vi "Loop.vi"(9 "Error Queue":refnum<queue>, 10 "Helper Loop Queue":refnum<queue>, 11 "Dev Actor Panel":refnum<class "Dev Panel.lvclass">) -> ()   [LabVIEW 2021, in "Dev Panel.lvclass"]
uses:
  Dev Panel.lvclass
  C:/git/jettl/src/Event Actor/Event Actor.lvclass
  Event Actor/Event Actor.lvclass
  Dev Panel.lvclass/Dev Panel.ctl
  Actor/Msgs/Teardown/Teardown Msg/Teardown Msg.lvclass
  C:/git/jettl/src/Actor/Msg/Msg.lvclass
  Msgs/Pop Up/Pop Up Msg/Pop Up Msg.lvclass
  Actor/Msgs/Merge Error/Merge Error Msg/Merge Error Msg.lvclass
panel:
  in  "Button":bool
  out "String Indicator":string
  in  "Pop Up":bool
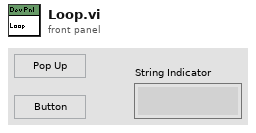
[diagram p1: front panel]
types:
  T1 = cluster{"Teardown":refnum<user-event>, "Pop Up":refnum<user-event>, "String Indicator":refnum<user-event>, "Button":refnum<user-event>}
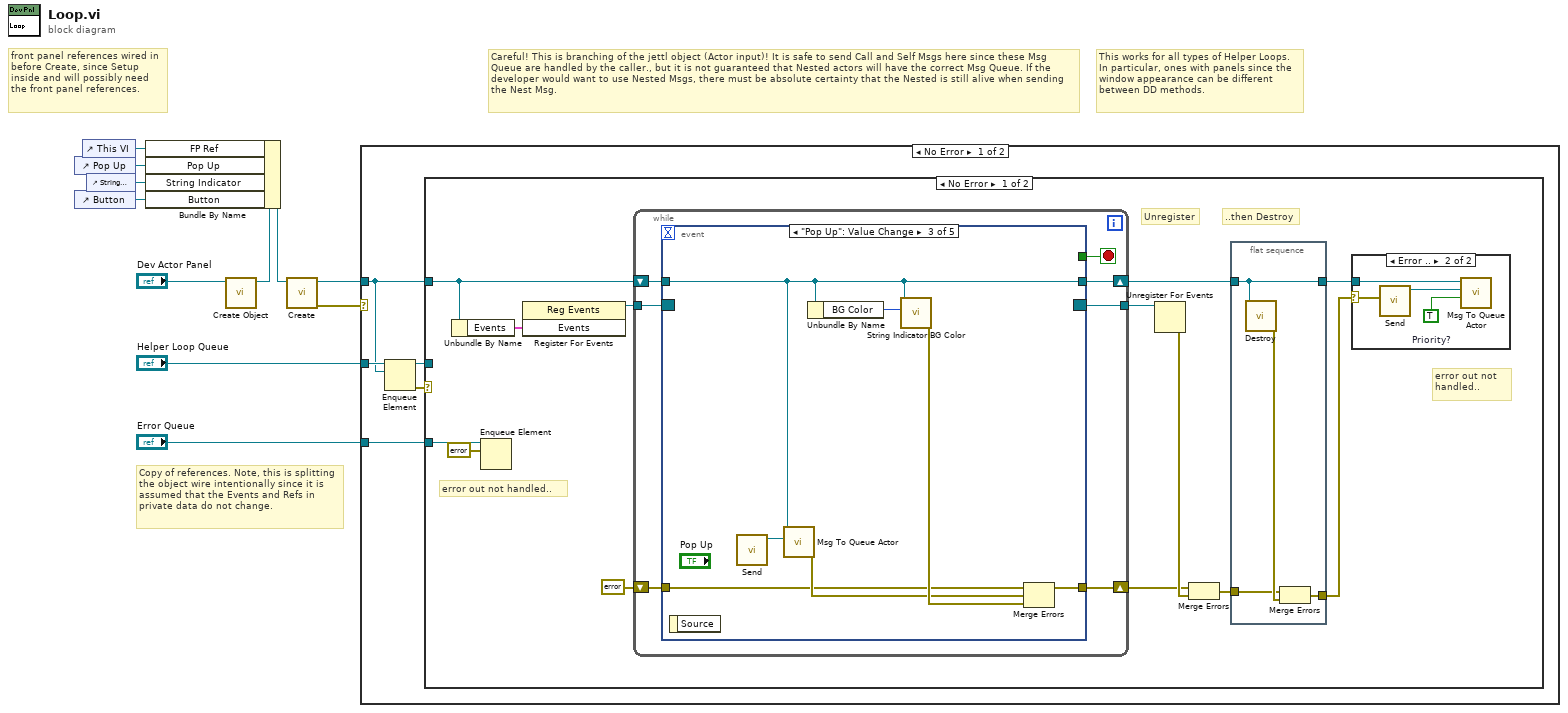
[diagram p0: block diagram]
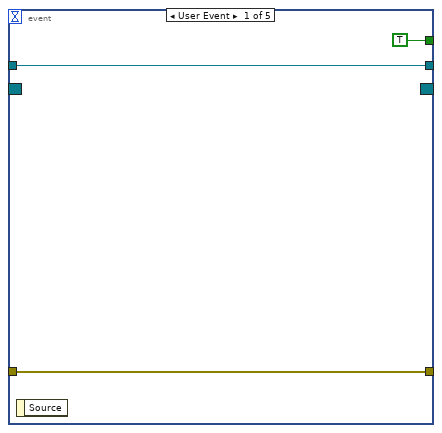
[diagram p3: hidden frame]
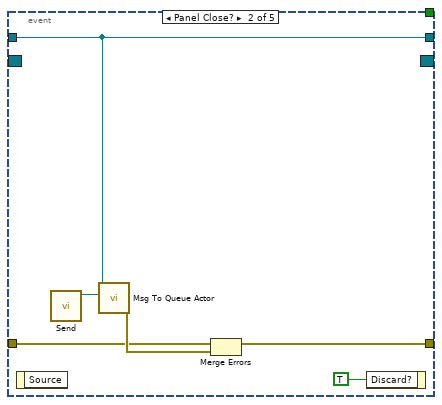
[diagram p4: hidden frame]
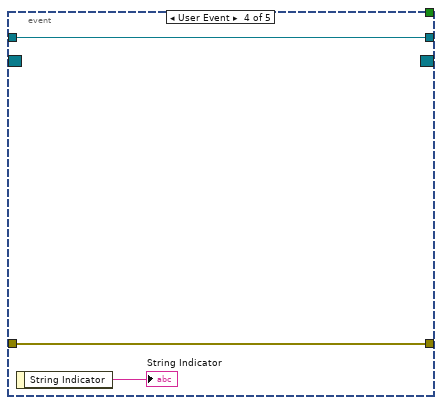
[diagram p5: hidden frame]
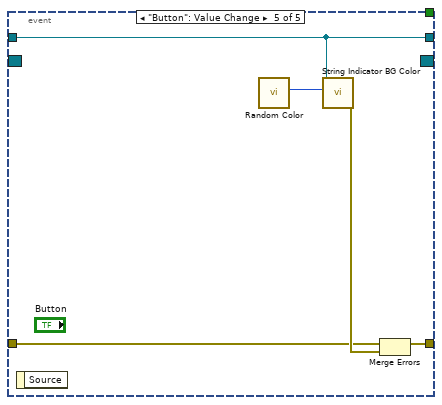
[diagram p6: hidden frame]
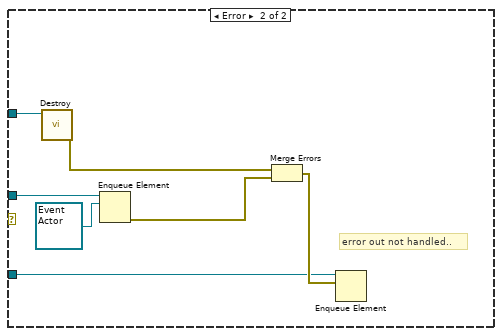
[diagram p7: hidden frame]
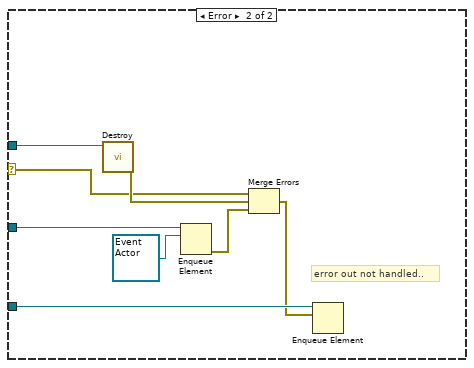
[diagram p8: hidden frame]
diagram:
  # "Copy of references. Note, this is splitting the object wire intentionally since it is assumed that the Events and Refs in private data do not change."
  # "front panel references wired in before Create, since Setup inside and will possibly need the front panel references."
  # "This works for all types of Helper Loops. In particular, ones with panels since the window appearance can be different between DD methods."
  # "Careful! This is branching of the jettl object (Actor input)! It is safe to send Call and Self Msgs here since these Msg Queue are handled by the caller., but it is not guaranteed that Nested actors will have the correct Msg Queue. If the developer would want to use Nested Msgs, there must be absolute certainty that the Nested is still alive when sending the Nest Msg."
  n1 = control-ref of="Pop Up"() -> (w9:refnum<vi>)
  n2 = control-ref of="Button"() -> (w8:refnum<vi>)
  n3 = control-ref of="This VI"() -> (w2:refnum<vi>)
  n4 = control-ref of="String Indicator"() -> (w10:refnum<vi>)
  n5 = call "Create Object.vi"("Dev Panel in"="Dev Actor Panel") -> ("Dev Panel out"=w3:refnum<class "Dev Panel.lvclass">)  [unwired: 10 in]
  n6 = Bundle By Name(cluster=w3, "FP Ref"=w2, "Pop Up"=w9, "String Indicator"=w10, "Button"=w8) -> (w4:refnum<class "Dev Panel.lvclass">)
  n7 = call "Create.vi"("Dev Actor Panel in"=w4) -> ("error out"=w11:errorcluster, "Dev Actor Panel out"=w5:refnum<class "Dev Panel.lvclass">)  [unwired: 9 in]
  n8 = case shown="No Error" w11 {
    selector: w11 -> [_ w81]
    tunnel: w5 -> [w14 w83]
    tunnel: "Error Queue" -> [w16 w80]
    tunnel: "Helper Loop Queue" -> [w15 w78]
    frame No Error {
      n9 = Enqueue Element(queue=w15, element=w14) -> (queue out=w12:refnum<queue>, error out=w13:errorcluster)  [unwired: 2 in, 1 out]
      n10 = case shown="No Error" w13 {
        tunnel: w16 -> [w20 w71]
        tunnel: w14 -> [w18 w69]
        tunnel: w12 -> [_ w70]
        frame No Error {
          # "error out not handled.."
          # "error out not handled.."
          # "..then Destroy"
          # "Unregister"
          n11 = Unbundle By Name(w18) -> ("Events"=w27:T1)
          n12 = Enqueue Element(queue=w20, element=errorcluster {"status"=FALSE, "code"=0, "source"=""}) -> ()  [unwired: 2 in, 3 out]
          n13 = register-events ("Main Register for Events")(w27) -> (reference out=w28:refnum<event-registration>)  [unwired: 2 in, 1 out]
          n14 = while {
            shift-right: [w41] -> w23
            shift-left: w18 -> [w40]
            tunnel: w28 -> [w44]
            tunnel: [w42] -> w29
            shift-right: [w39] -> w24
            shift-left: errorcluster {"status"=FALSE, "code"=0, "source"=""} ("error out") -> [w38]
            stop <- w43 stop-if-true
            n15 = event "UI Events" shown="[2] \"Pop Up\": Value Change" {
              selector: w44 -> [_ _ _ _ _]
              dyn-events: [_ _ _ _ _] -> w42
              timeout: _ -> [_ _ _ _ _]
              tunnel: [TRUE _ _ _ _] -> w43
              tunnel: [w46 w51 w57 w63 w68] -> w41
              tunnel: w40 -> [w46 w51 w57 w63 w68]
              tunnel: [w45 w52 w60 w62 w67] -> w39
              tunnel: w38 -> [w45 w48 w54 w62 w65]
              event User Event {
                n16 = event-data() -> ()  [unwired: 1 in, 1 out]
              }
              event Panel Close? {
                n17 = event-data() -> ()  [unwired: 1 in, 1 out]
                n18 = call "Send.vi"() -> ("Teardown Msg out"=w50:refnum<class "Teardown Msg.lvclass">)  [unwired: 11 in]
                n19 = call-dynamic "Msg To Queue Actor.vi"("Msg"=w50, "Dev Panel in"=w51) -> ("error out"=w49:errorcluster)  [unwired: 9 in]
                n20 = Merge Errors(w48, w49) -> (w52:errorcluster)
                n21 = event-data("Discard?"=TRUE) -> ()  [unwired: 1 in, 1 out]
              }
              event "Pop Up": Value Change {
                n22 = event-data() -> ()  [unwired: 1 in, 1 out]
                n23 = call "Send.vi"() -> ("Pop Up Msg out"=w56:refnum<class "Pop Up Msg.lvclass">)  [unwired: 11 in]
                n24 = call-dynamic "Msg To Queue Actor.vi"("Msg"=w56, "Dev Panel in"=w57) -> ("error out"=w55:errorcluster)  [unwired: 9 in]
                n25 = Unbundle By Name(w57) -> ("BG Color"=w58:u32)
                n26 = call "String Indicator BG Color.vi"("BG Color"=w58, "Dev Panel in"=w57) -> ("error out"=w59:errorcluster)  [unwired: 9 in]
                n27 = Merge Errors(w54, w55, w59) -> (w60:errorcluster)
              }
              event User Event {
                n28 = event-data() -> ("String Indicator"=→"String Indicator":string)  [unwired: 1 in]
              }
              event "Button": Value Change {
                n29 = event-data() -> ()  [unwired: 1 in, 1 out]
                n30 = call "Random Color.vi"() -> ("Color"=w64:u32)  [unwired: 11 in]
                n31 = call "String Indicator BG Color.vi"("BG Color"=w64, "Dev Panel in"=w68) -> ("error out"=w66:errorcluster)  [unwired: 9 in]
                n32 = Merge Errors(w65, w66) -> (w67:errorcluster)
              }
            }
          }
          n33 = Unregister For Events(event registration refnum=w29) -> (error out=w25:errorcluster)  [unwired: 1 in]
          n34 = Merge Errors(w24, w25) -> (w22:errorcluster)
          n35 = flat-sequence {
            tunnel: w23 -> [w34]
            tunnel: [w37] -> w21
            tunnel: w22 -> [w35]
            tunnel: [w34] -> w17
            frame #0 {
              n36 = call "Destroy.vi"("Dev Actor Panel in"=w34) -> ("error out"=w36:errorcluster)  [unwired: 10 in]
              n37 = Merge Errors(w35, w36) -> (w37:errorcluster)
            }
          }
          n38 = case shown="Error .." w21 {
            selector: w21 -> [_ w33]
            tunnel: w17 -> [_ w32]
            frame No Error {
            }
            frame Error {
              w30 = TRUE  # Priority?
              n39 = call "Send.vi"("Error"=w33) -> ("Merge Error Msg out"=w31:refnum<class "Merge Error Msg.lvclass">)  [unwired: 10 in]
              n40 = call-dynamic "Msg To Queue Actor.vi"("Priority?"=w30, "Msg"=w31, "Dev Panel in"=w32) -> ()  [unwired: 8 in, 1 out]
            }
          }
        }
        frame Error {
          # "error out not handled.."
          n41 = call "Destroy.vi"("Dev Actor Panel in"=w69) -> ("error out"=w75:errorcluster)  [unwired: 10 in]
          n42 = Enqueue Element(queue=w70, element=refnum<class "Event Actor.lvclass"> refnum) -> (error out=w72:errorcluster)  [unwired: 2 in, 2 out]
          n43 = Merge Errors(w75, w72) -> (w74:errorcluster)
          n44 = Enqueue Element(queue=w71, element=w74) -> ()  [unwired: 2 in, 3 out]
        }
      }
    }
    frame Error {
      # "error out not handled.."
      n45 = call "Destroy.vi"("Dev Actor Panel in"=w83) -> ("error out"=w82:errorcluster)  [unwired: 10 in]
      n46 = Enqueue Element(queue=w78, element=refnum<class "Event Actor.lvclass"> refnum) -> (error out=w76:errorcluster)  [unwired: 2 in, 2 out]
      n47 = Merge Errors(w81, w82, w76) -> (w79:errorcluster)
      n48 = Enqueue Element(queue=w80, element=w79) -> ()  [unwired: 2 in, 3 out]
    }
  }
